vi "Renew Container Lease.vi"(8 "error in (no error)":errorcluster, 9 "Lease ID":string, 10 "Container":string, 11 "Azure Session in":refnum<class "Session.lvclass">) -> (0 "error out":errorcluster, 3 "Azure Session out":refnum<class "Session.lvclass">)   [LabVIEW 2015, in "NI_Azure_Blob.lvlib"]
doc: "Renew an existing lease on a container."
uses:
  NI_Azure_Blob.lvlib
  Core/Session/Session.lvclass
  Core/Name Value Pair.ctl
  Lease Action.ctl
  Core/Session/Session.lvclass/Session.ctl
  Core/Session/Write Request Headers.vi
  Core/Session/Write Request Parameters.vi
  Core/Session/Write HTTP Verb.vi
  Core/Session/Write URL Suffix.vi
  Core/NI_Azure_Core.lvlib
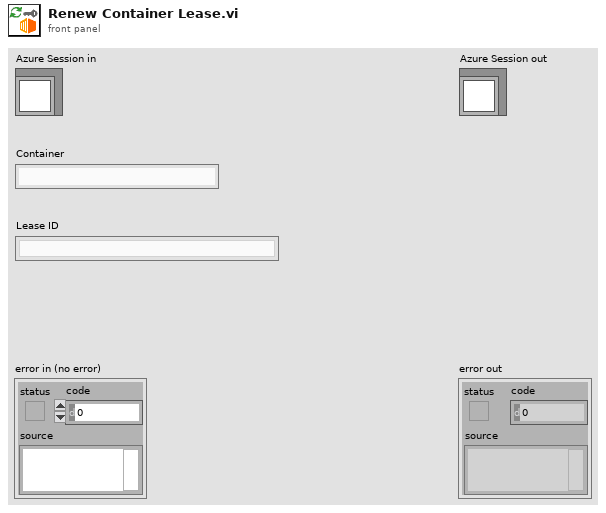
[diagram p1: front panel]
types:
  T1 = typedef "NI_Azure_Blob.lvlib/Lease Action.ctl" = enum16{"acquire", "renew", "change", "release", "break"}
  T2 = typedef "NI_Azure_Core.lvlib/Name Value Pair.ctl" = cluster{"name":string, "value":string}
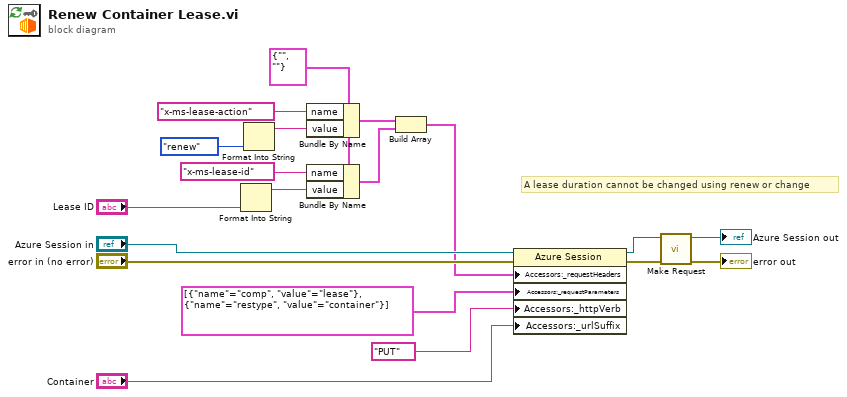
[diagram p0: block diagram]
diagram:
  w12 = T2 {"name"="", "value"=""} ("Cluster")
  # "A lease duration cannot be changed using renew or change"
  n1 = Format Into String("Lease ID") -> (resulting string=w10:string)  [unwired: 3 in, 1 out]
  n2 = Format Into String(Lease_Action."renew" ("Lease action")) -> (resulting string=w14:string)  [unwired: 3 in, 1 out]
  n3 = Bundle By Name(cluster=w12, "name"="x-ms-lease-action" ("header"), "value"=w14) -> (w16:T2)
  n4 = Bundle By Name(cluster=w12, "name"="x-ms-lease-id" ("header"), "value"=w10) -> (w9:T2)
  n5 = Build Array(w16, w9) -> (w3:T2[])
  n6 = property class="Azure Session"(reference="Azure Session in", error in="error in (no error)", "Accessors:_requestHeaders"=w3, "Accessors:_requestParameters"=T2[] [{"name"="comp", "value"="lease"}, {"name"="restype", "value"="container"}] ("request parameters"), "Accessors:_httpVerb"="PUT" ("HTTP-Verb"), "Accessors:_urlSuffix"="Container") -> (reference out=w5:refnum<class "Session.lvclass">, error out=w7:errorcluster)
  n7 = call "Make Request.vi"("error in (no error)"=w7, "Session in"=w5) -> ("error out"=→"error out":errorcluster, "Session out"=→"Azure Session out":refnum<class "Session.lvclass">)  [unwired: 7 in, 1 out]
